vi "DPT TC Panel Write.vi"(11 "TC Panel 1 Out":T1[][](array[typedef])) -> (3 "Array":string[][](array[string]))   [LabVIEW 2016]
doc: "Organize information to be written to config file."
uses:
  Type Definitions/DPT Channel Label.ctl
  Utility/Custom Pallet Controls/Custom Pallet String.ctl
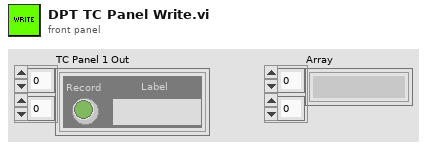
[diagram p1: front panel]
types:
  T1 = typedef "DPT Channel Label.ctl" = cluster{"Label":T2, "Record":bool, "Index":u32, "Channel":string}
  T2 = typedef "Custom Pallet String.ctl" = string
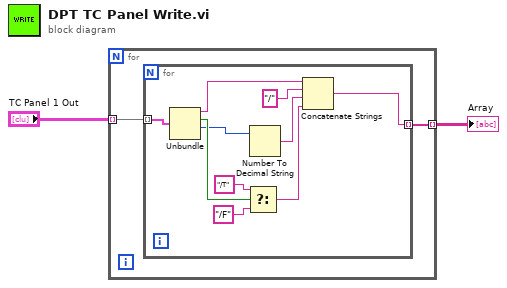
[diagram p0: block diagram]
diagram:
  n1 = for {
    tunnel: "TC Panel 1 Out" -> [w4] mode=indexing
    tunnel: [w3] -> w1 mode=indexing
    n2 = for {
      tunnel: w4 -> [w14] mode=indexing
      tunnel: [w9] -> w3 mode=indexing
      n3 = Unbundle(w14) -> ("Label"=w13:T2, "Record"=w8:bool, "Index"=w6:u32)  [unwired: 1 out]
      n4 = Select(t="/T" ("string"), s=w8, f="/F" ("string")) -> (s? t:f=w10:string)
      n5 = Number To Decimal String(number=w6) -> (decimal integer string=w5:string)  [unwired: 1 in]
      n6 = Concatenate Strings(w13, "/" ("string"), w5, w10) -> (w9:string)
    }
  }
  "Array" <- w1
